vi "robot kol.vi"   [LabVIEW 2016]
uses:
  <vilib>/LabVIEW Interface for Arduino/LabVIEW Interface for Arduino.lvlib
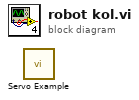
[diagram p0: block diagram]
diagram:
  n1 = call <vilib>:"Servo Example.vi"() -> ()  [unwired: 1 in]
